vi "AudioStreamer.IsOpen.vi"() -> (0 "success":bool)   [LabVIEW 2020]
panel:
  out "error out":errorcluster
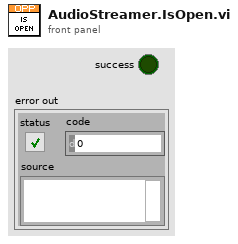
[diagram p1: front panel]
types:
  T1 = enum32{"Bad", "Idle", "Run top level", "Running"}
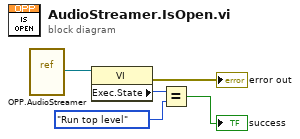
[diagram p0: block diagram]
diagram:
  n1 = vi-ref "OPP.AudioStreamer.vi"() -> (w3:refnum<vi>)
  n2 = property class="VI"(reference=w3) -> (error out=→"error out":errorcluster, "Exec.State"=w4:T1)  [unwired: 1 in, 1 out]
  n3 = Equal?(x=w4, y=T1."Run top level" ("Execution:State")) -> (x = y?=→"success":bool)
